vi "RunScript.vi"(8 "error in":errorcluster, 10 "script":string, 11 "Python":T1) -> (0 "error out":errorcluster, 2 "Tx":string, 3 "Python":T1)   [LabVIEW 2020]
uses:
  PythonCtrl.ctl
  _subs/Processors.ctl
panel:
  out "Reply":string
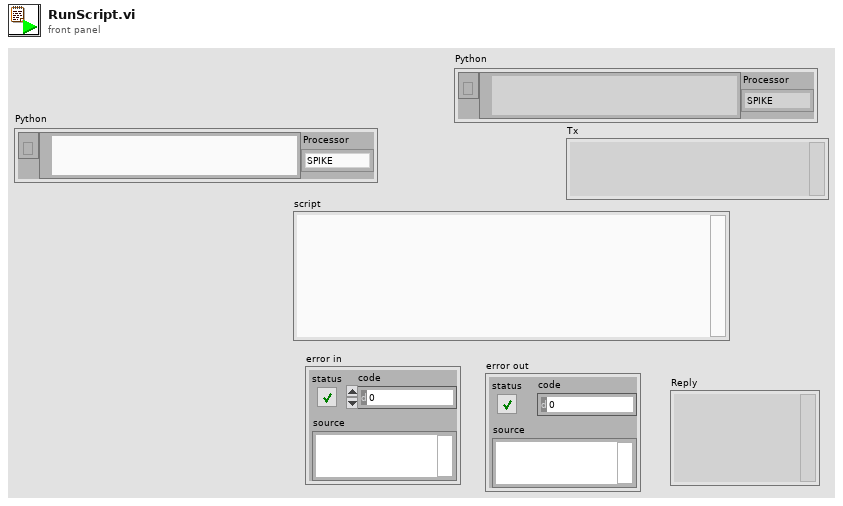
[diagram p1: front panel]
types:
  T1 = typedef "PythonCtrl.ctl" = cluster{"session":refnum<k35>, "PyPath":path, "Processor":T2}
  T2 = typedef "Processors.ctl" = enum16{"SPIKE", "Pi", "Pi_ssh", "OpenMV"}
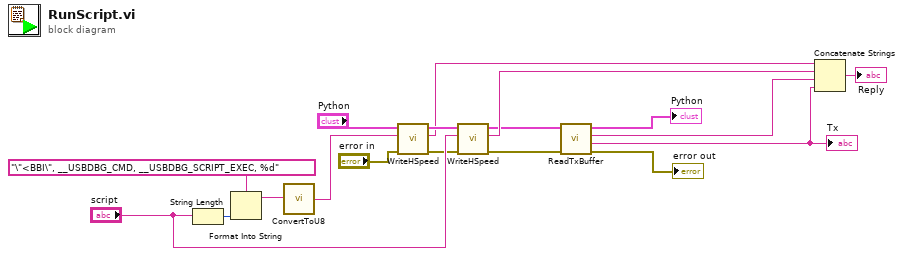
[diagram p0: block diagram]
diagram:
  n1 = String Length(string="script") -> (length=w17:i32)
  n2 = Format Into String(format string="\"<BBI\", __USBDBG_CMD, __USBDBG_SCRIPT_EXEC, %d" ("write buffer"), w17) -> (resulting string=w6:string)  [unwired: 2 in, 1 out]
  n3 = call "ConvertToU8.vi"("struct"=w6) -> ("Binary"=w5:string)
  n4 = call "WriteHSpeed.vi"("error in"="error in", "write buffer"=w5, "Python"="Python") -> ("error out"=w13:errorcluster, "read buffer"=w11:string, "Python"=w16:T1)  [unwired: 6 in]
  n5 = call "WriteHSpeed.vi"("error in"=w13, "write buffer"="script", "Python"=w16) -> ("error out"=w3:errorcluster, "read buffer"=w12:string, "Python"=w2:T1)  [unwired: 6 in]
  n6 = call "ReadTxBuffer.vi"("error in"=w3, "Python"=w2) -> ("error out"=→"error out":errorcluster, "Tx Buffer"=w4:string, "Tx Buffer Len"=w9:string, "Python"=→"Python":T1)  [unwired: 6 in]
  "Tx" <- w4
  n7 = Concatenate Strings(w11, w12, w9, w4) -> (→"Reply":string)
